vi "get millisecond tick count.vi"(11 "error in":errorcluster) -> (1 "tick count (ms)":u32, 3 "error out":errorcluster)   [LabVIEW 2013]
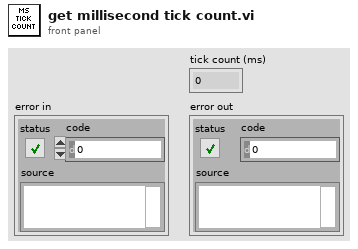
[diagram p1: front panel]
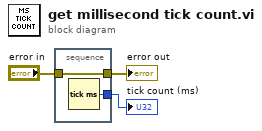
[diagram p0: block diagram]
diagram:
  n1 = stacked-sequence {
    tunnel: "error in" -> [w5]
    tunnel: [w5] -> w2
    tunnel: [w4] -> w1
    frame #0 {
      n2 = Tick Count (ms)() -> (millisecond timer value=w4:u32)
    }
  }
  "error out" <- w2
  "tick count (ms)" <- w1
